vi "DataTreeCtrlFM Test.vi"() -> ()   [LabVIEW 2018]
uses:
  ctl/FMstateMachineEnum.ctl
  DataTreeCtrl.lvclass
panel:
  in  "deleteIndexes":u8[](array[numeric])
  out "outputArr":string[][](array[string])
  in  "getState":bool
  in  "delete":bool
  out "error out":errorcluster
  in  "error in (no error)":errorcluster
  in  "tdmsFilePath in":path=path "D:/msdata python/C60_KEExam2.tdms"
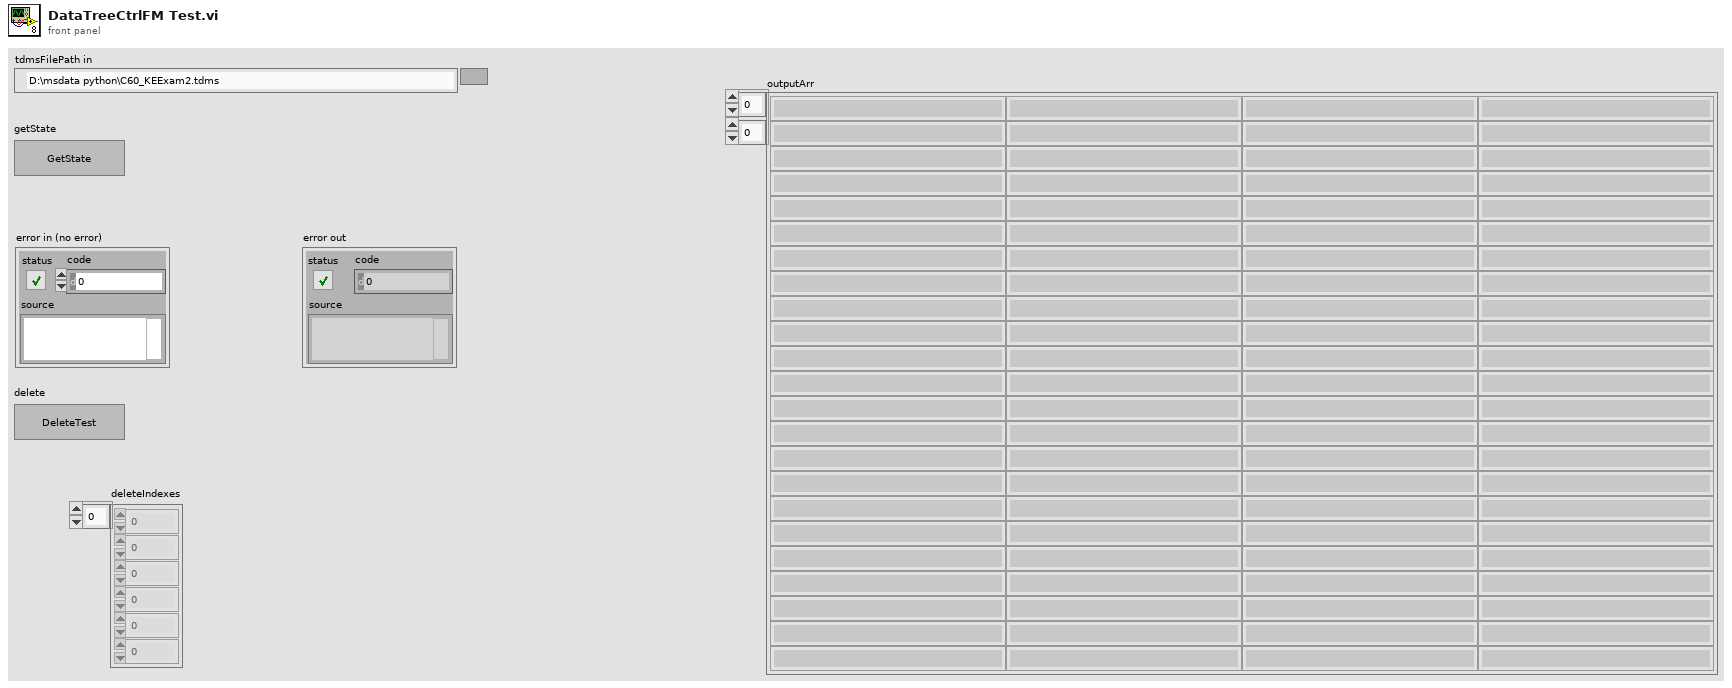
[diagram p1: front panel]
types:
  T1 = typedef "FMstateMachineEnum.ctl" = enum16{"none", "init", "openTDMS", "closeTDMS", "getDataList", "getDataInfo", "getTimeStamp", "getCurrPath", "getComment", "overwriteComment", "readData", "deleteData", "moveData"}
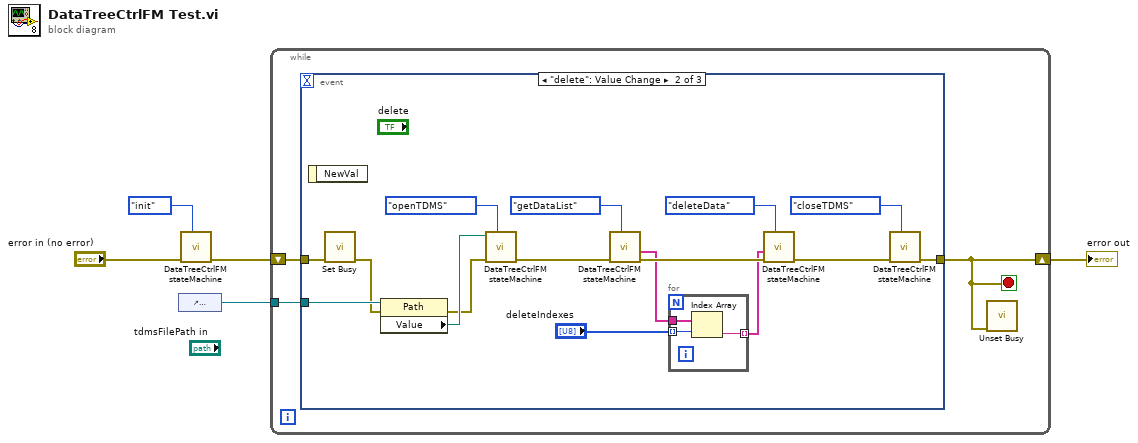
[diagram p0: block diagram]
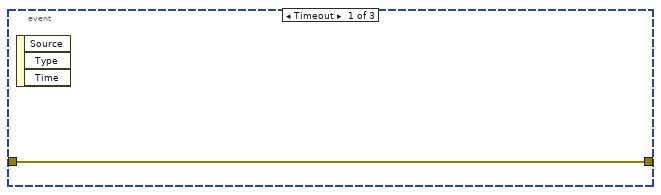
[diagram p2: hidden frame]
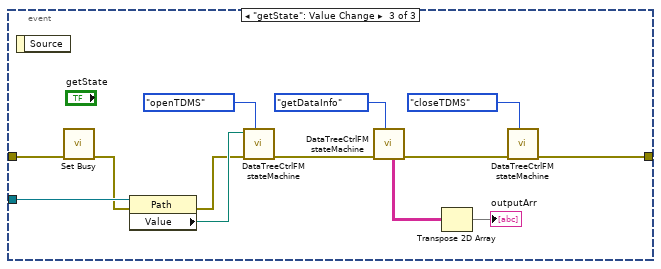
[diagram p3: hidden frame]
diagram:
  n1 = control-ref of="tdmsFilePath in"() -> (w2:refnum<vi>)
  n2 = call "DataTreeCtrlFM stateMachine.vi"("Func"=FMstateMachineEnum."init", "error in (no error)"="error in (no error)") -> ("error out"=w3:errorcluster)  [unwired: 4 in, 5 out]
  n3 = while {
    shift-right: [w6] -> w1
    shift-left: w3 -> [w8]
    tunnel: w2 -> [w7]
    stop <- w6 stop-if-true
    n4 = event shown="[1] \"delete\": Value Change" {
      selector: _ -> [_ _ _]
      dyn-events: _ -> [_ _ _]
      timeout: _ -> [_ _ _]
      tunnel: [w9 w16 w29] -> w6
      tunnel: w8 -> [w9 w14 w34]
      tunnel: w7 -> [_ w20 w37]
      event Timeout {
        n5 = event-data() -> ()  [unwired: 1 in, 3 out]
      }
      event "delete": Value Change {
        n6 = event-data() -> ()  [unwired: 1 in, 1 out]
        n7 = call <vilib>:"Set Busy.vi"("error in (no error)"=w14) -> ("error out"=w12:errorcluster)  [unwired: 9 in, 1 out]
        n8 = property class="Path"(reference=w20, error in=w12) -> (error out=w13:errorcluster, "Value"=w19:path)  [unwired: 1 out]
        n9 = call "DataTreeCtrlFM stateMachine.vi"("Func"=FMstateMachineEnum."openTDMS", "error in (no error)"=w13, "tdmsFilePath in"=w19) -> ("error out"=w21:errorcluster)  [unwired: 3 in, 5 out]
        n10 = call "DataTreeCtrlFM stateMachine.vi"("Func"=FMstateMachineEnum."getDataList", "error in (no error)"=w21) -> ("error out"=w23:errorcluster, "dataList"=w15:string[])  [unwired: 4 in, 4 out]
        n11 = for {
          tunnel: w15 -> [w28]
          tunnel: "deleteIndexes" -> [w27] mode=indexing
          tunnel: [w26] -> w10 mode=indexing
          n12 = Index Array(array=w28, index=w27) -> (element=w26:string)
        }
        n13 = call "DataTreeCtrlFM stateMachine.vi"("Func"=FMstateMachineEnum."deleteData", "error in (no error)"=w23, "multiDatasName"=w10) -> ("error out"=w17:errorcluster)  [unwired: 3 in, 5 out]
        n14 = call "DataTreeCtrlFM stateMachine.vi"("Func"=FMstateMachineEnum."closeTDMS", "error in (no error)"=w17) -> ("error out"=w16:errorcluster)  [unwired: 4 in, 5 out]
      }
      event "getState": Value Change {
        n15 = event-data() -> ()  [unwired: 1 in, 1 out]
        n16 = call <vilib>:"Set Busy.vi"("error in (no error)"=w34) -> ("error out"=w33:errorcluster)  [unwired: 9 in, 1 out]
        n17 = property class="Path"(reference=w37, error in=w33) -> (error out=w32:errorcluster, "Value"=w36:path)  [unwired: 1 out]
        n18 = call "DataTreeCtrlFM stateMachine.vi"("Func"=FMstateMachineEnum."openTDMS", "error in (no error)"=w32, "tdmsFilePath in"=w36) -> ("error out"=w39:errorcluster)  [unwired: 3 in, 5 out]
        n19 = call "DataTreeCtrlFM stateMachine.vi"("Func"=FMstateMachineEnum."getDataInfo", "error in (no error)"=w39) -> ("error out"=w30:errorcluster, "outputArr"=w40:string[][])  [unwired: 4 in, 4 out]
        n20 = Transpose 2D Array(2D array=w40) -> (transposed array=→"outputArr":string[][])
        n21 = call "DataTreeCtrlFM stateMachine.vi"("Func"=FMstateMachineEnum."closeTDMS", "error in (no error)"=w30) -> ("error out"=w29:errorcluster)  [unwired: 4 in, 5 out]
      }
    }
    n22 = call <vilib>:"Unset Busy.vi"("error in (no error)"=w6) -> ()  [unwired: 10 in, 1 out]
  }
  "error out" <- w1
